vi "Post New Media Tweet (LabVIEW Picture Type) - Finite.vi"() -> ()   [LabVIEW 2011]
doc: "This example posts a tweet and LabVIEW picture data type to twitter."
uses:
  i3-twitter.lvlib
panel:
  in  "LabVIEW Picture":picture
  in  "Tweet":string
  in  "Consumer Secret":string
  in  "Consumer Key":string
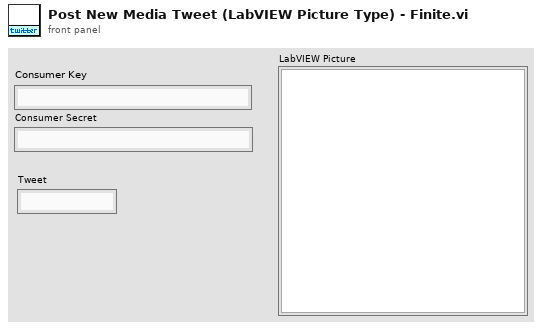
[diagram p1: front panel]
types:
  T1 = typedef "i3-oauth.lvlib/Credentials.ctl" = cluster{"Token":string, "Secret":string}
  T2 = typedef "i3-twitter.lvlib/Twitter Handle.ctl" = cluster{"OAuth Credentials":T3, "since ID":string, "max ID":string, "Screen Name":string}
  T3 = typedef "i3-oauth.lvlib/OAuth Handle.ctl" = cluster{"Signature Method":T4, "Version":string, "Client":T1, "Access":T1}
  T4 = typedef "i3-oauth.lvlib/Signature Method.ctl" = enum16{"HMAC-MD5", "HMAC-SHA1", "HMAC-SHA224", "HMAC-SHA256", "HMAC-SHA384", "HMAC-SHA512"}
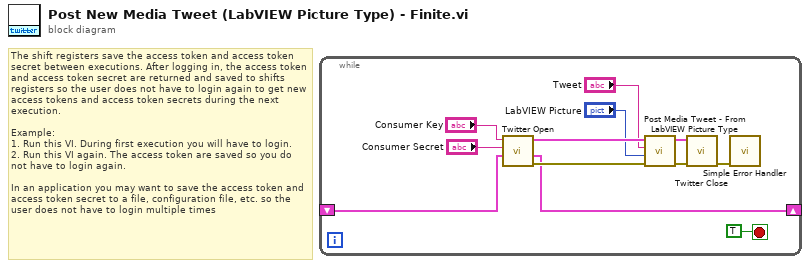
[diagram p0: block diagram]
diagram:
  # "The shift registers save the access token and access token secret between executions. After logging in, the access token and access token secret are returned and saved to shifts registers so the user does not have to login again to get new access tokens and access token secrets during the next execution.\n\nExample:\n1. Run this VI. During first execution you will have to login.\n2. Run this VI again. The access token are saved so you do not have to login again.\n\nIn an application you may want to save the access token and access token secret to a file, configuration file, etc. so the user does not have to login multiple times"
  n1 = while {
    shift-right: [w2] -> _
    shift-left: _ -> [w1]
    stop <- TRUE stop-if-true
    n2 = call "Twitter Open.vi"("Access Credentials (in)"=w1, "Consumer Secret"="Consumer Secret", "Consumer Key"="Consumer Key") -> ("error out"=w12:errorcluster, "Access Credentials (out)"=w2:T1, "Twitter Handle Out"=w10:T2)  [unwired: 6 in]
    n3 = call "Post Media Tweet - From LabVIEW Picture Type.vi"("error in"=w12, "LabVIEW Picture Type"="LabVIEW Picture", "Tweet"="Tweet", "Twitter Handle In"=w10) -> ("error out"=w11:errorcluster, "Twitter Handle Out"=w9:T2)  [unwired: 6 in]
    n4 = call "Twitter Close.vi"("error in"=w11, "Twitter Handle In"=w9) -> ("error in"=w5:errorcluster)  [unwired: 9 in]
    n5 = call <vilib>:"Simple Error Handler.vi"("error in (no error)"=w5) -> ()  [unwired: 4 in, 5 out]
  }
